vi "Get All Channel groups.vi"(8 "error in (no error)":errorcluster, 11 "FPGA Device in":refnum<class "FPGA Device.lvclass">) -> (0 "error out":errorcluster, 1 "Channel Groups":refnum<class "Channel group.lvclass">[](array[class]), 2 "names":string[](array[string]), 3 "FPGA Device out":refnum<class "FPGA Device.lvclass">)   [LabVIEW 2016, in "FPGA RM Shared API.lvlib" / "FPGA Device.lvclass"]
uses:
  FPGA Device.lvclass
  Channel Group/Channel group.lvclass
  FPGA Device.lvclass/FPGA Device.ctl
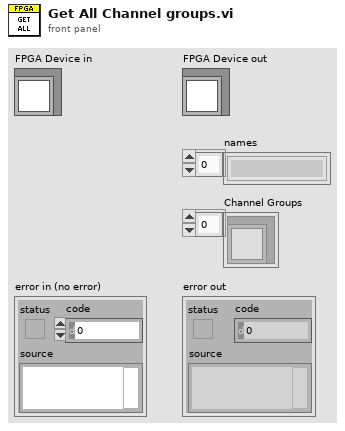
[diagram p1: front panel]
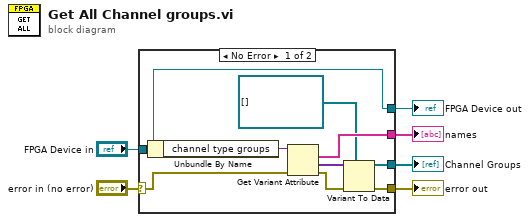
[diagram p0: block diagram]
diagram:
  n1 = case shown="No Error" "error in (no error)" {
    selector: "error in (no error)" -> [w8 w17]
    tunnel: [w11 w17] -> w5
    tunnel: [w15 w16] -> w3
    tunnel: "FPGA Device in" -> [w15 w16]
    tunnel: [w13 _] -> w2
    tunnel: [w9 _] -> w1
    frame No Error {
      n2 = Unbundle By Name(w15) -> ("channel type groups"=w14:variant)
      n3 = Get Variant Attribute(Variant=w14, error in=w8) -> (names=w13:string[], values=w12:variant[], error out=w7:errorcluster)  [unwired: 2 in, 1 out]
      n4 = Variant To Data(error in=w7, type=refnum<class "Channel group.lvclass">[] [] ("Array"), Variant=w12) -> (data=w9:refnum<class "Channel group.lvclass">[], error out=w11:errorcluster)
    }
    frame Error {
    }
  }
  "error out" <- w5
  "FPGA Device out" <- w3
  "names" <- w2
  "Channel Groups" <- w1
